vi "TEST_Eurotherm.vi"() -> ()   [LabVIEW 2017]
uses:
  MODBUS_EUROTHERM P116_485/Eurotherm_2023_Module.ctl
  MODBUS_EUROTHERM P116_485/Address.ctl
panel:
  out "Numeric":i32
  out "Valid":bool
  out "Eurotherm":T1
  in  "stop":bool
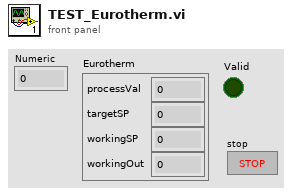
[diagram p1: front panel]
types:
  T1 = cluster{"processVal":dbl, "targetSP":dbl, "workingSP":dbl, "workingOut":dbl}
  T2 = typedef "SECADO_comms--Cluster.ctl" = cluster{"Eurotherm":refnum<visa-resource-name>, "CDT":bool, "Agilent":refnum<visa-resource-name>, "AGL":bool, "#Dec":u16}
  T3 = typedef "Address.ctl" = enum16{"Add 1", "Add 2", "Add 3", "Add 4", "Add 5", "Add 6", "Add 10", "Add 11", "Add 12", "Add 13"}
  T4 = typedef "Eurotherm_2023_Module.ctl" = enum16{"Initialize", "Write setpoint", "Read data", "Write ramp rate", "Set constante proporcional", "Set constante integral", "Set constante diferencial", "Set ouput limit LOW", "Set ouput limit HIGH", "Shutdown"}
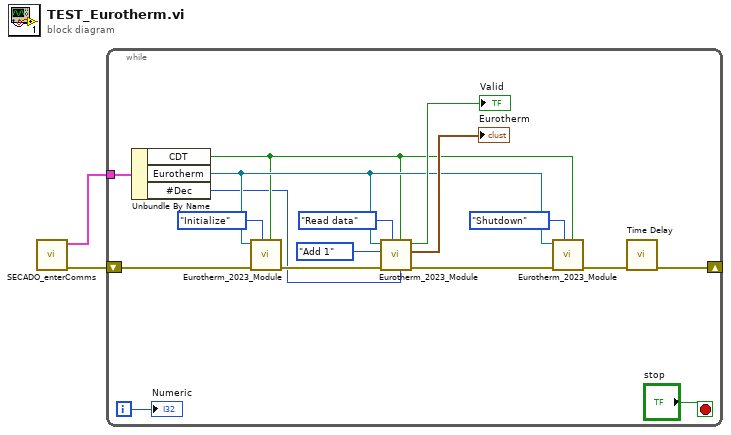
[diagram p0: block diagram]
diagram:
  n1 = call "SECADO_enterComms.vi"() -> ("error out"=w2:errorcluster, "Comunicaciones"=w1:T2)  [unwired: 9 in, 1 out]
  n2 = while {
    shift-right: [w5] -> _
    shift-left: w2 -> [w10]
    tunnel: w1 -> [w9]
    i -> [w3]
    stop <- "stop" stop-if-true
    n3 = Unbundle By Name(w9) -> ("CDT"=w7:bool, "Eurotherm"=w8:refnum<visa-resource-name>, "#Dec"=w6:u16)
    n4 = call "Eurotherm_2023_Module.vi"("Eurotherm (T:Enable)"=w7, "Command"=Eurotherm_2023_Module."Initialize", "error in (no error)"=w10, "VISA resource name"=w8) -> ("error out"=w17:errorcluster)  [unwired: 5 in, 2 out]
    n5 = call "Eurotherm_2023_Module.vi"("Decimales"=w6, "Eurotherm (T:Enable)"=w7, "Command"=Eurotherm_2023_Module."Read data", "error in (no error)"=w17, "Address"=Address."Add 1", "VISA resource name"=w8) -> ("error out"=w18:errorcluster, "Eurotherm"=→"Eurotherm":T1, "Valid"=→"Valid":bool)  [unwired: 3 in]
    n6 = call "Eurotherm_2023_Module.vi"("Eurotherm (T:Enable)"=w7, "Command"=Eurotherm_2023_Module."Shutdown", "error in (no error)"=w18, "VISA resource name"=w8) -> ("error out"=w4:errorcluster)  [unwired: 5 in, 2 out]
    n7 = call "Time Delay"("error in (no error)"=w4) -> ("error out"=w5:errorcluster)  [unwired: 10 in]
    "Numeric" <- w3
  }
